vi "To Serial Form.vi"(6 "Serial Version":T1, 10 "Serializer in":refnum<class "Serializer.lvclass">, 11 "Humidity Control in":refnum<class "Humidity Control.lvclass">) -> (0 "error out":errorcluster, 2 "Serializer out":refnum<class "Serializer.lvclass">, 3 "Humidity Control out":refnum<class "Humidity Control.lvclass">)   [LabVIEW 2012, in "Humidity Control.lvclass"]
uses:
  Humidity Control.lvclass
  <userlib>/Serialization/Serializable/Serializable.lvclass
  <userlib>/Serialization/Serializable/Insert Double.vi
  <userlib>/Serialization/Serializable/Insert Single.vi
  <userlib>/Serialization/Serializer/Serializer.lvclass
  <userlib>/Serialization/Serialization Common/Serial Version.ctl
  <userlib>/Serialization/Serialization Common/Serialization Common.lvlib
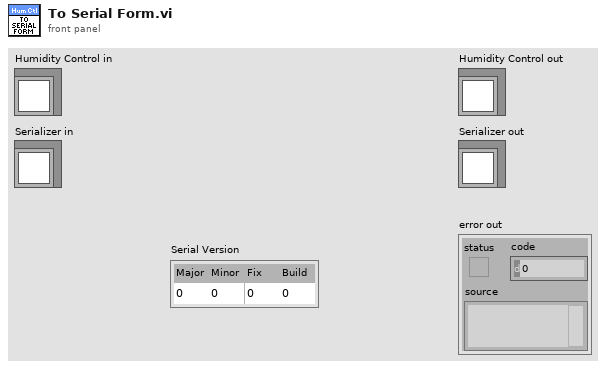
[diagram p1: front panel]
types:
  T1 = typedef "Serialization Common.lvlib/Serial Version.ctl" = cluster{"Major":u16, "Minor":u16, "Fix":u16, "Build":u16}
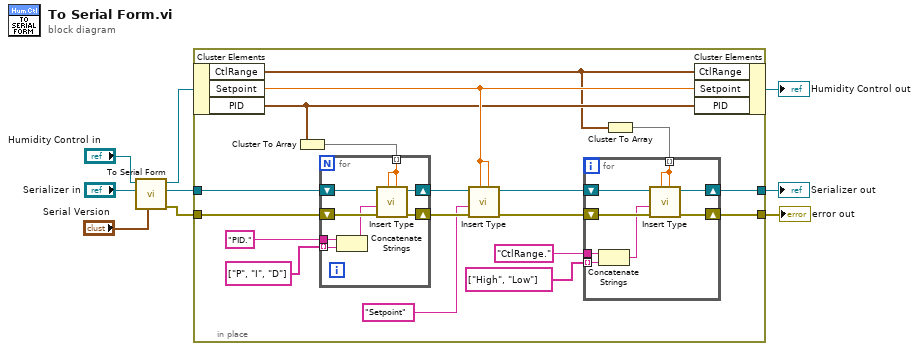
[diagram p0: block diagram]
diagram:
  n1 = call-parent "To Serial Form.vi"("Serial Version"="Serial Version", "Serializer in"="Serializer in", "Serializable in"="Humidity Control in") -> ("error out"=w4:errorcluster, "Serializer out"=w5:refnum<class "Serializer.lvclass">, "Serializable out"=w6:refnum<class "Humidity Control.lvclass">)  [unwired: 6 in]
  n2 = in-place {
    in-place-border: w5 -> [w27]
    in-place-border: w4 -> [w26]
    in-place-border: [w19] -> w3
    in-place-border: [w18] -> w1
    n3 = in-place-cluster #1(w6) -> ("CtlRange"=w13:cluster{"high":dbl, "low":dbl}, "Setpoint"=w25:sgl, "PID"=w17:cluster{"P":dbl, "I":dbl, "D":dbl})
    n4 = Cluster To Array(cluster=w17) -> (array=w16:dbl[])
    n5 = for {
      tunnel: w16 -> [w39] mode=indexing
      shift-right: [w41] -> w24
      shift-left: w27 -> [w43]
      tunnel: string[] ["P", "I", "D"] -> [w38] mode=indexing
      tunnel: "PID." -> [w37]
      shift-right: [w40] -> w23
      shift-left: w26 -> [w42]
      n6 = Concatenate Strings(w37, w38) -> (w36:string)
      n7 = call-poly <userlib>:"Insert Type.vi"("Double"=w39, "Default Value"=w39, "error in (no error)"=w42, "Name"=w36, "Serializer in"=w43) -> ("error out"=w40:errorcluster, "Serializer out"=w41:refnum<class "Serializer.lvclass">)  [unwired: 5 in]
    }
    n8 = call-poly <userlib>:"Insert Type.vi"("Double"=w25, "Default Value"=w25, "error in (no error)"=w23, "Name"="Setpoint", "Serializer in"=w24) -> ("error out"=w20:errorcluster, "Serializer out"=w21:refnum<class "Serializer.lvclass">)  [unwired: 5 in]
    n9 = Cluster To Array(cluster=w13) -> (array=w12:dbl[])
    n10 = for {
      tunnel: w12 -> [w31] mode=indexing
      shift-right: [w33] -> w19
      shift-left: w21 -> [w35]
      shift-right: [w32] -> w18
      shift-left: w20 -> [w34]
      tunnel: string[] ["High", "Low"] -> [w30] mode=indexing
      tunnel: "CtlRange." -> [w29]
      n11 = Concatenate Strings(w29, w30) -> (w28:string)
      n12 = call-poly <userlib>:"Insert Type.vi"("Double"=w31, "Default Value"=w31, "error in (no error)"=w34, "Name"=w28, "Serializer in"=w35) -> ("error out"=w32:errorcluster, "Serializer out"=w33:refnum<class "Serializer.lvclass">)  [unwired: 5 in]
    }
    n13 = in-place-cluster #1("CtlRange"=w13, "Setpoint"=w25, "PID"=w17) -> (→"Humidity Control out":refnum<class "Humidity Control.lvclass">)
  }
  "error out" <- w1
  "Serializer out" <- w3
